vi "Sampling.vi"() -> ()   [LabVIEW 2009]
doc: "For an aliased, uncorrupted replica to appear at baseband without being distorted itself, Fs > Passband Bandwidth, and the carrier frequency must be an integer multiple of the sampling rate. Only for real spectra. See 'Undersampling Complex Signals' section in included document for explanation.\n\nNote: Magnitude may be slightly distorted at lower sampling rates due to windowing / other signal conditioning effects inherent to LabVIEW. To reiterate: Sampling like so: f[n] = f(nTs), where Ts is the sampling period, results in spectral scaling by fs, the sampling frequency, and periodic repetition of the spectra in frequency with a period equal to your sampling frequency."
uses:
  <vilib>/Analysis/4window.llb/windowTd.ctl
  <vilib>/measure/maspectr.llb/FFT Spectrum (Mag-Phase) for 1 Chan.vi
  <vilib>/Analysis/2dsp.llb/Resample (constant to constant,single -channel).vi
  <vilib>/Analysis/NI_AALBase.lvlib
  <vilib>/measure/NI_MABase.lvlib
  <vilib>/Analysis/NI_AALPro.lvlib
  <vilib>/measure/NI_MAPro.lvlib
panel:
  in  "Real / Complex Spectra":bool=TRUE
  out "error out":errorcluster
  in  "Carrier Amplitude":dbl=1.0
  in  "Tone / Spectra":bool=TRUE
  in  "Carrier Frequency":dbl=200000000.0 format="%#_6p"
  in  "Signal Passband Bandwidth":dbl=100000000.0 format="%#_6p"
  in  "Sampling Rate":dbl=550000000.0 format="%#_6p"
  out "Magnitude Spectrum of output of A/D converter sampling at Sampling Rate":cluster{"f0":dbl, "df":dbl, "magnitude":dbl[]}(graph)={"f0"=0.0, "df"=100127.4349171673, "magnitude"=[]}
  out "Input Signal Magnitude Spectrum":cluster{"f0":dbl, "df":dbl, "magnitude":dbl[]}(graph)={"f0"=0.0, "df"=100000.00000000001, "magnitude"=[]}
  in  "Duration (Seconds)":dbl=1e-05
  # "*For more information on each a control, please see the description for that control"
  # "Configuration"
  # "Aliasing"
  # "Frequency of continuous\ninput to sampler"
  # "Input Frequency"
  # "Fs/2"
  # "Fs"
  # "2Fs"
  # "3Fs"
  # "Apparent Frequency of Sampled Signal"
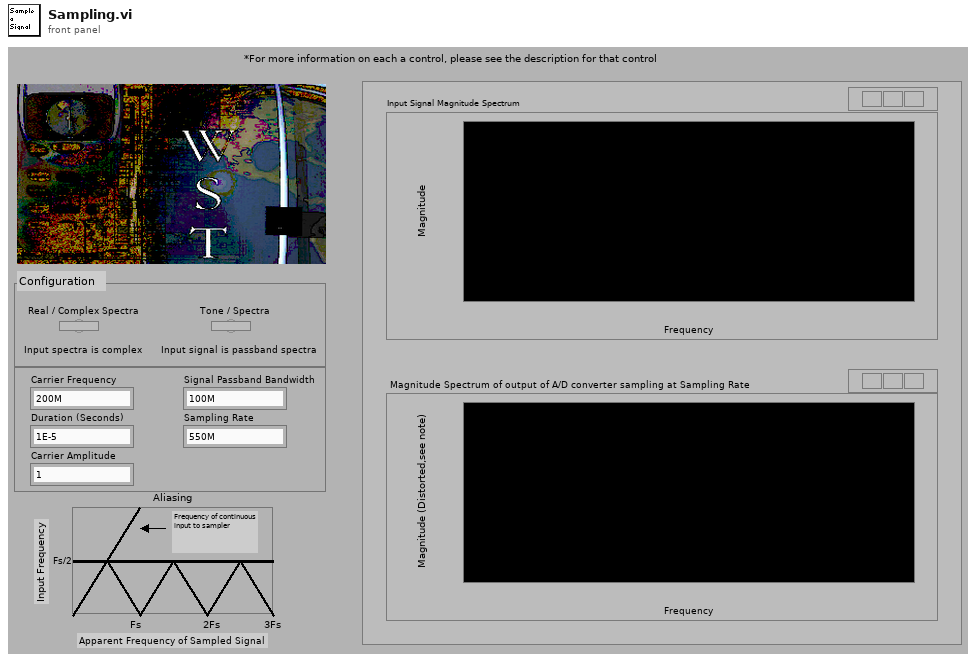
[diagram p1: front panel]
types:
  T1 = typedef "NI_AALPro.lvlib/windowTd.ctl" = u32
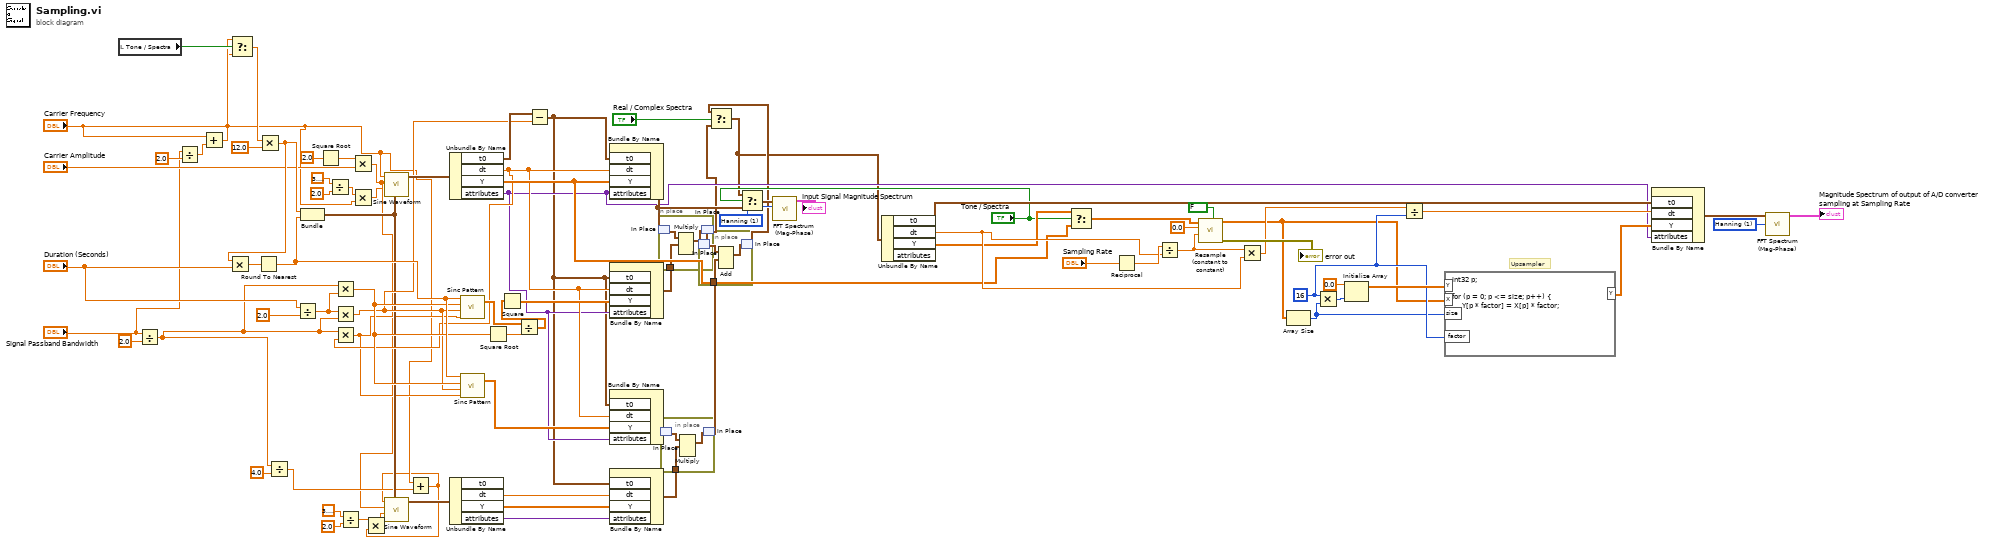
[diagram p0: block diagram]
diagram:
  w52 = 16 ("x")
  w74 = T1 1 items=["Rectangle"=0, "Hanning"=1, "Hamming"=2, "Blackman-Harris"=3, "Exact Blackman"=4, "Blackman"=5, "Flat Top"=6, "4 Term B-Harris "=7, "7 Term B-Harris"=8, "Low Sidelobe"=9, "Blackman Nuttall"=11, "Triangle"=30, "Kaiser"=60, "Dolph-Chebyshev"=61, "Gaussian"=62] ("window")
  w76 = T1 1 items=["Rectangle"=0, "Hanning"=1, "Hamming"=2, "Blackman-Harris"=3, "Exact Blackman"=4, "Blackman"=5, "Flat Top"=6, "4 Term B-Harris "=7, "7 Term B-Harris"=8, "Low Sidelobe"=9, "Blackman Nuttall"=11, "Triangle"=30, "Kaiser"=60, "Dolph-Chebyshev"=61, "Gaussian"=62] ("window")
  # "Upsampler"
  n1 = local read "Tone / Spectra"() -> (w65:bool)
  n2 = Divide(x="Signal Passband Bandwidth", y=2.0) -> (x/y=w26:dbl)
  n3 = Divide(x="Signal Passband Bandwidth", y=2.0) -> (x/y=w80:dbl)
  n4 = Add(x="Carrier Frequency", y=w80) -> (x+y=w62:dbl)
  n5 = Select(t=w62, s=w65, f="Carrier Frequency") -> (s? t:f=w64:dbl)
  n6 = Multiply(x=w64, y=12.0) -> (x*y=w78:dbl)
  n7 = Multiply(x=w78, y="Duration (Seconds)") -> (x*y=w83:dbl)
  n8 = Round To Nearest(number=w83) -> (nearest integer value=w35:dbl)
  n9 = Divide(x=w26, y=4.0) -> (x/y=w25:dbl)
  n10 = Divide(x="Duration (Seconds)", y=2.0 ("amplitude")) -> (x/y=w42:dbl)
  n11 = Bundle(w78, w35) -> (w29:cluster{dbl, dbl})  [unwired: 1 in]
  n12 = Square Root(x=2.0) -> (sqrt(x)=w60:dbl)
  n13 = Divide(x=3.141592653589793, y=2.0 ("phase")) -> (x/y=w13:dbl)
  n14 = Multiply(x=w26, y=w42) -> (x*y=w34:dbl)
  n15 = Multiply(x=w42, y=w26) -> (x*y=w33:dbl)
  n16 = Divide(x=3.141592653589793, y=2.0 ("phase")) -> (x/y=w8:dbl)
  n17 = Multiply(x=w60, y="Carrier Amplitude") -> (x*y=w24:dbl)
  n18 = Multiply(x=w13, y="Carrier Frequency") -> (x*y=w11:dbl)
  n19 = call <vilib>:"Sine Waveform.vi"("sampling info"=w29, "phase"=w11, "amplitude"=w24, "frequency"="Carrier Frequency") -> ("signal out"=w47:waveform(dbl))  [unwired: 6 in, 1 out]
  n20 = Add(x="Carrier Frequency", y=w25) -> (x+y=w7:dbl)
  n21 = Multiply(x=w8, y=w7) -> (x*y=w6:dbl)
  n22 = call <vilib>:"Sine Waveform.vi"("sampling info"=w29, "phase"=w6, "amplitude"=w24, "frequency"=w7) -> ("signal out"=w23:waveform(dbl))  [unwired: 6 in, 1 out]
  n23 = Unbundle By Name(w47) -> ("t0"=w46:timestamp, "dt"=w31:dbl, "Y"=w45:dbl[], "attributes"=w30:variant)
  n24 = Multiply(x=w26, y=w31) -> (x*y=w28:dbl)
  n25 = Unbundle By Name(w23) -> ("dt"=w21:dbl, "Y"=w19:dbl[], "attributes"=w20:variant)  [unwired: 1 out]
  n26 = call <vilib>:"Sinc Pattern.vi"("delta t"=w28, "delay"=w33, "amplitude"=w34, "samples"=w35) -> ("Sinc Pattern"=w38:dbl[])  [unwired: 1 out]
  n27 = call <vilib>:"Sinc Pattern.vi"("delta t"=w28, "delay"=w33, "amplitude"=w34, "samples"=w35) -> ("Sinc Pattern"=w32:dbl[])  [unwired: 1 out]
  n28 = Square Root(x=w34) -> (sqrt(x)=w39:dbl)
  n29 = Divide(x=w38, y=w39) -> (x/y=w36:dbl[])
  n30 = Square(x=w36) -> (x^2=w37:dbl[])
  n31 = Subtract(x=w46, y=w33) -> (x-y=w22:timestamp)
  n32 = Bundle By Name("t0"=w22, "dt"=w31, "Y"=w45, "attributes"=w30) -> (w44:waveform(dbl))  [unwired: 1 in]
  n33 = Bundle By Name("t0"=w22, "dt"=w31, "Y"=w37, "attributes"=w30) -> (w82:waveform(dbl))  [unwired: 1 in]
  n34 = Bundle By Name("t0"=w22, "dt"=w31, "Y"=w32, "attributes"=w30) -> (w17:waveform(dbl))  [unwired: 1 in]
  n35 = Bundle By Name("t0"=w22, "dt"=w21, "Y"=w19, "attributes"=w20) -> (w16:waveform(dbl))  [unwired: 1 in]
  n36 = in-place {
    in-place-border: w82 -> [w88]
    n37 = in-place-match #1(w44) -> (w87:waveform(dbl))
    n38 = Multiply(1:w88, 2:w87) -> (0:w86:waveform(dbl))  [unwired: 1 in, 1 out]
    n39 = in-place-match #1(w86) -> (w5:waveform(dbl))
  }
  n40 = in-place {
    in-place-border: w16 -> [w89]
    n41 = in-place-match #2(w17) -> (w90:waveform(dbl))
    n42 = Multiply(1:w89, 2:w90) -> (0:w91:waveform(dbl))  [unwired: 1 in, 1 out]
    n43 = in-place-match #2(w91) -> (w18:waveform(dbl))
  }
  n44 = in-place {
    in-place-border: w18 -> [w94]
    n45 = in-place-match #3(w5) -> (w93:waveform(dbl))
    n46 = Add(1:w94, 2:w93) -> (0:w92:waveform(dbl))  [unwired: 1 in, 1 out]
    n47 = in-place-match #3(w92) -> (w3:waveform(dbl))
  }
  n48 = Select(t=w3, s="Real / Complex Spectra", f=w5) -> (s? t:f=w2:waveform(dbl))
  n49 = Select(t=w2, s="Tone / Spectra", f=w44) -> (s? t:f=w61:waveform(dbl))
  n50 = call-poly <vilib>:"FFT Spectrum (Mag-Phase).vi"("window"=w76, "time signal"=w61) -> ("magnitude"=→"Input Signal Magnitude Spectrum":cluster{"f0":dbl, "df":dbl, "magnitude":dbl[]})  [unwired: 5 in, 4 out]
  n51 = Unbundle By Name(w2) -> ("t0"=w73:timestamp, "dt"=w69:dbl, "Y"=w66:dbl[])  [unwired: 1 out]
  n52 = Select(t=w66, s="Tone / Spectra", f=w45) -> (s? t:f=w67:dbl[])
  n53 = Reciprocal(x="Sampling Rate") -> (1/x=w70:dbl)
  n54 = Divide(x=w70, y=w69) -> (x/y=w72:dbl)
  n55 = call-poly <vilib>:"Resample (constant to constant).vi"("anti-aliasing?"=FALSE, "dt"=w72, "delay"=0.0, "X"=w67) -> ("error out"=→"error out":errorcluster, "Y"=w49:dbl[])  [unwired: 5 in, 1 out]
  n56 = Multiply(x=w72, y=w69) -> (x*y=w50:dbl)
  n57 = Array Size(array=w49) -> (size(s)=w51:i32)
  n58 = Multiply(x=w52, y=w51) -> (x*y=w54:i32)
  n59 = Initialize Array(0.0 ("element"), w54) -> (w53:dbl[])
  n60 = Divide(x=w50, y=w52) -> (x/y=w56:dbl)
  n61 = formula code="int32 p;\n\nfor (p = 0; p <= size; p++) {\n     Y[p * factor] = X[p] * factor;\n}"("X"=w49, "size"=w51, "factor"=w52, "Y"=w53) -> ("Y"=w48:dbl[])
  n62 = Bundle By Name("t0"=w73, "dt"=w56, "Y"=w48, "attributes"=w30) -> (w71:waveform(dbl))  [unwired: 1 in]
  n63 = call-poly <vilib>:"FFT Spectrum (Mag-Phase).vi"("window"=w74, "time signal"=w71) -> ("magnitude"=→"Magnitude Spectrum of output of A/D converter sampling at Sampling Rate":cluster{"f0":dbl, "df":dbl, "magnitude":dbl[]})  [unwired: 5 in, 4 out]
